vi "Weather Station UI.vi"() -> ()   [LabVIEW 2018]
doc: "This is the main VI in the Weather Station project. It contains the user interface for a temperature warning system. Temperature is retrieved every half second; data is logged when a warning has occurred."
uses:
  Supporting Files/Station States.ctl
  Supporting Files/Weather Data.ctl
  Instance           2 26Saved   Weather Station UI .vi
panel:
  in  "Station Number":string="A12345"
  in  "Operator Name":string="Leonardo DaVinci"
  out "Warning":string
  in  "Lower Limit":dbl=20.0
  in  "Upper Limit":dbl=30.0
  in  "Stop Button":bool
  out "Temperature History":dbl(graph)
  # "Temperature Ranges (C)"
  # "Freeze"
  # "Heat \nStroke"
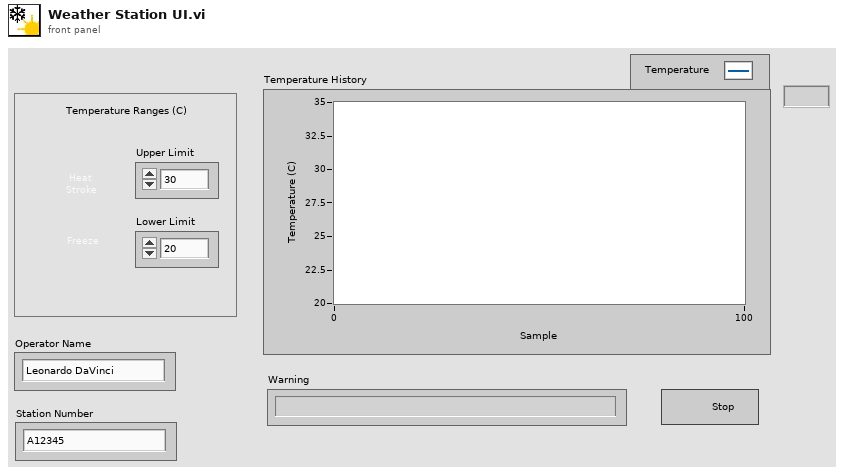
[diagram p1: front panel]
types:
  T1 = typedef "Weather Data.ctl" = cluster{"Current Temperature":dbl, "Max Temperature":dbl, "Min Temperature":dbl, "Temperature Warning?":bool, "Temperature Warning Text":string}
  T2 = typedef "Station States.ctl" = enum16{"Acquisition", "Analysis", "Data Log", "Time Check"}
  T3 = enum16{"open", "replace", "create", "open or create", "replace or create", "replace or create with confirmation"}
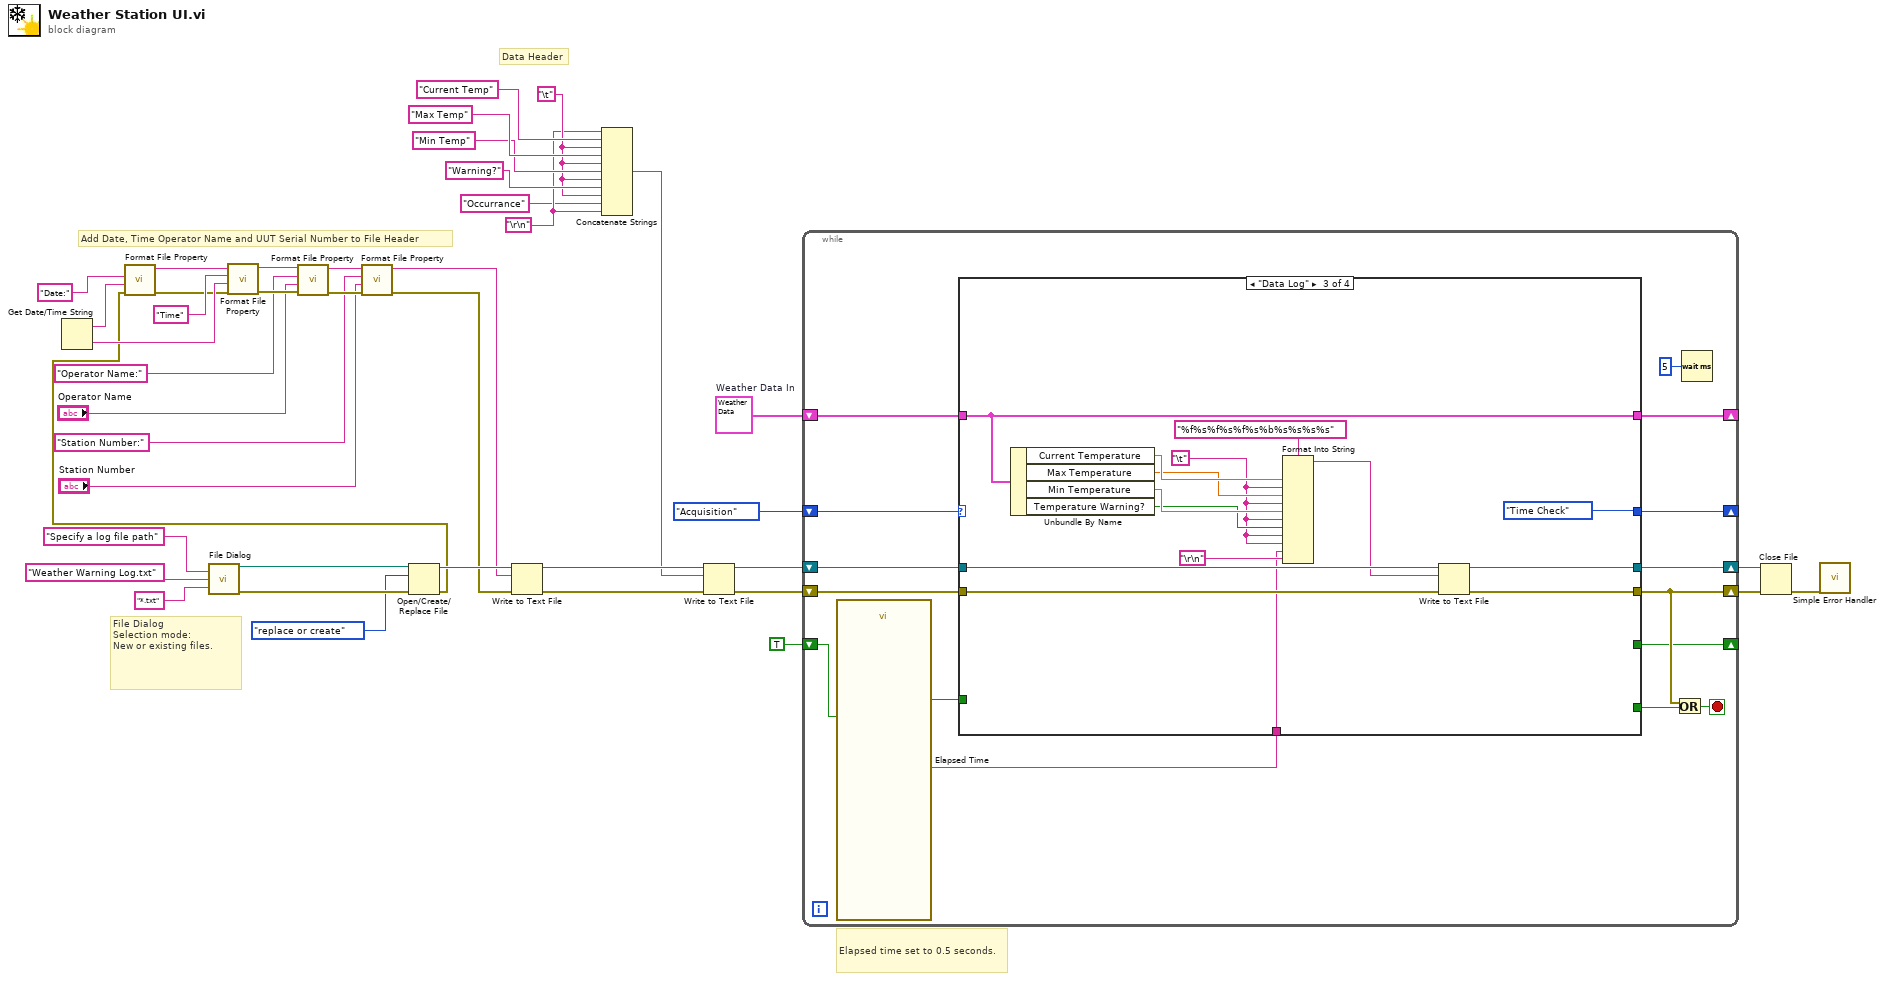
[diagram p0: block diagram]
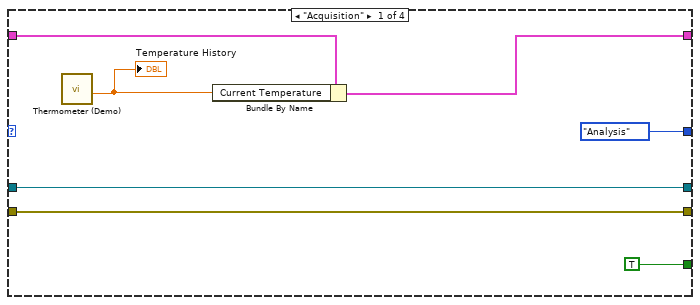
[diagram p2: hidden frame]
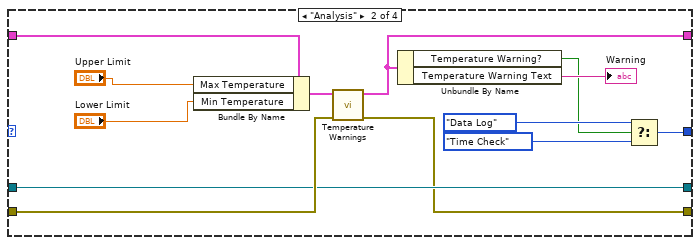
[diagram p3: hidden frame]
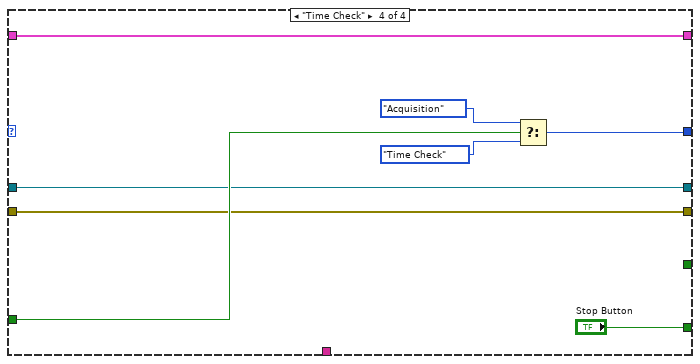
[diagram p4: hidden frame]
diagram:
  w2 = "\r\n"
  w3 = "\t"
  w29 = T1 {"Current Temperature"=0.0, "Max Temperature"=0.0, "Min Temperature"=0.0, "Temperature Warning?"=FALSE, "Temperature Warning Text"="No Warning"}  # Weather Data In
  # "Data Header"
  # "Elapsed time set to 0.5 seconds."
  # "Add Date, Time Operator Name and UUT Serial Number to File Header"
  # "File Dialog\nSelection mode:\nNew or existing files."
  n1 = Get Date/Time String() -> (date string=w26:string, time string=w23:string)  [unwired: 3 in]
  n2 = call "File Dialog"("prompt"="Specify a log file path", "default name"="Weather Warning Log.txt", "pattern (all files)"="*.txt" ("pattern label")) -> ("selected path"=w36:path, "error out"=w33:errorcluster)  [unwired: 9 in, 2 out]
  n3 = Open/Create/Replace File(file path (use dialog)=w36, error in=w33, operation (0:open)=T3."replace or create") -> (refnum out=w37:refnum<file>, error out=w11:errorcluster)  [unwired: 3 in, 1 out]
  n4 = call "Format File Property.vi"("Error In"=w11, "File Property Value"=w26, "File Property Name"="Date:") -> ("Error Out"=w20:errorcluster, "String out"=w24:string)  [unwired: 7 in]
  n5 = call "Format File Property.vi"("Error In"=w20, "File Property Value"=w23, "File Property Name"="Time", "String in"=w24) -> ("Error Out"=w21:errorcluster, "String out"=w22:string)  [unwired: 6 in]
  n6 = call "Format File Property.vi"("Error In"=w21, "File Property Value"="Operator Name", "File Property Name"="Operator Name:", "String in"=w22) -> ("Error Out"=w19:errorcluster, "String out"=w18:string)  [unwired: 6 in]
  n7 = call "Format File Property.vi"("Error In"=w19, "File Property Value"="Station Number", "File Property Name"="Station Number:", "String in"=w18) -> ("Error Out"=w10:errorcluster, "String out"=w13:string)  [unwired: 6 in]
  n8 = Write to Text File(file (use dialog)=w37, text=w13, error in=w10) -> (refnum out=w28:refnum<file>, error out=w12:errorcluster)  [unwired: 1 in, 1 out]
  n9 = Concatenate Strings(w2, "Current Temp" ("string"), w3, "Max Temp" ("string"), w3, "Min Temp" ("string"), w3, "Warning?" ("string"), w3, "Occurrance" ("string"), w2) -> (w4:string)
  n10 = Write to Text File(file (use dialog)=w28, text=w4) -> (refnum out=w9:refnum<file>)  [unwired: 2 in, 2 out]
  n11 = while {
    shift-right: [w49] -> w41
    shift-left: w12 -> [w56]
    shift-right: [w54] -> w40
    shift-left: w9 -> [w53]
    shift-right: [w44] -> _
    shift-left: TRUE ("stop") -> [w51]
    shift-right: [w45] -> _
    shift-left: Station_States."Acquisition" -> [w48]
    shift-right: [w46] -> _
    shift-left: w29 -> [w47]
    stop <- w55 stop-if-true
    n12 = call "Elapsed Time"("Reset"=w51) -> ("Present Text"=w42:string, "Time has Elapsed"=w50:bool)  [unwired: 11 in, 6 out]
    n13 = case shown="\"Data Log\"" w48 {
      tunnel: [w62 w70 w85 w93] -> w49
      tunnel: w56 -> [w62 w72 w82 w93]
      tunnel: [w63 w71 w84 w94] -> w54
      tunnel: w53 -> [w63 w71 w83 w94]
      tunnel: w50 -> [_ _ _ w96]
      tunnel: w47 -> [w60 w76 w91 w92]
      tunnel: [w59 w69 w91 w92] -> w46
      tunnel: [Station_States."Analysis" w65 Station_States."Time Check" w99] -> w45
      tunnel: [TRUE _ _ _] -> w44
      tunnel: [_ _ _ "Stop Button"] -> w43
      tunnel: w42 -> [_ _ w78 _]
      frame "Acquisition" {
        n14 = call "Thermometer (Demo).vi"() -> ("Temperature Value"=w61:dbl)  [unwired: 11 in]
        "Temperature History" <- w61
        n15 = Bundle By Name(cluster=w60, "Current Temperature"=w61) -> (w59:T1)
      }
      frame "Analysis" {
        n16 = Bundle By Name(cluster=w76, "Max Temperature"="Upper Limit", "Min Temperature"="Lower Limit") -> (w73:T1)
        n17 = call "Temperature Warnings.vi"("Error In"=w72, "Weather Data In"=w73) -> ("Error Out"=w70:errorcluster, "Weather Data Out"=w69:T1)  [unwired: 8 in]
        n18 = Unbundle By Name(w69) -> ("Temperature Warning?"=w64:bool, "Temperature Warning Text"=→"Warning":string)
        n19 = Select(t=Station_States."Data Log", s=w64, f=Station_States."Time Check") -> (s? t:f=w65:T2)
      }
      frame "Data Log" {
        w77 = "\t"
        n20 = Unbundle By Name(w91) -> ("Current Temperature"=w89:dbl, "Max Temperature"=w88:dbl, "Min Temperature"=w87:dbl, "Temperature Warning?"=w86:bool)
        n21 = Format Into String(format string="%f%s%f%s%f%s%b%s%s%s%s", w89, w77, w88, w77, w87, w77, w86, w77, w77, w78, "\r\n") -> (resulting string=w81:string)  [unwired: 2 in, 1 out]
        n22 = Write to Text File(file (use dialog)=w83, text=w81, error in=w82) -> (refnum out=w84:refnum<file>, error out=w85:errorcluster)  [unwired: 1 in, 1 out]
      }
      frame "Time Check" {
        n23 = Select(t=Station_States."Acquisition", s=w96, f=Station_States."Time Check") -> (s? t:f=w99:T2)
      }
    }
    n24 = Or(x=w49, y=w43) -> (x .or. y?=w55:bool)
    n25 = Wait (ms)(milliseconds to wait=u32 5 ("y")) -> ()  [unwired: 1 out]
  }
  n26 = Close File(refnum=w40, error in=w41) -> (error out=w39:errorcluster)  [unwired: 1 out]
  n27 = call <vilib>:"Simple Error Handler.vi"("error in (no error)"=w39) -> ()  [unwired: 4 in, 5 out]
